vi "test_Open TCP connection using Initialize node.vi"(8 "error in (no error)":errorcluster, 11 "TestCase in":refnum<class "Ethernet Protocol Tests.lvclass">) -> (0 "error out":errorcluster, 3 "TestCase out":refnum<class "Ethernet Protocol Tests.lvclass">)   [LabVIEW 2019, in "Ethernet Protocol Tests.lvclass"]
uses:
  Ethernet Protocol Tests.lvclass
  TCP/TCP.lvclass
  TCP/TCP.lvclass/TCP.ctl
  Constants.vi
  <vilib>/addons/_JKI Toolkits/VI Tester/TestCase.llb/TestCase.lvclass
  C:/Program Files (x86)/National Instruments/LabVIEW 2019/vi.lib/addons/_JKI Toolkits/VI Tester/TestCase.llb/TestCase.lvclass
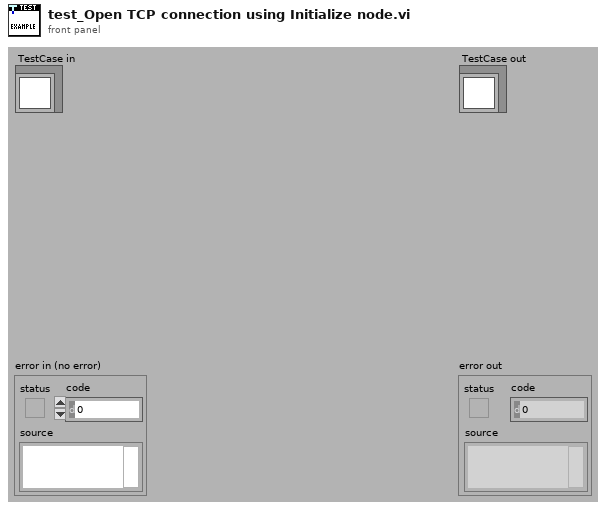
[diagram p1: front panel]
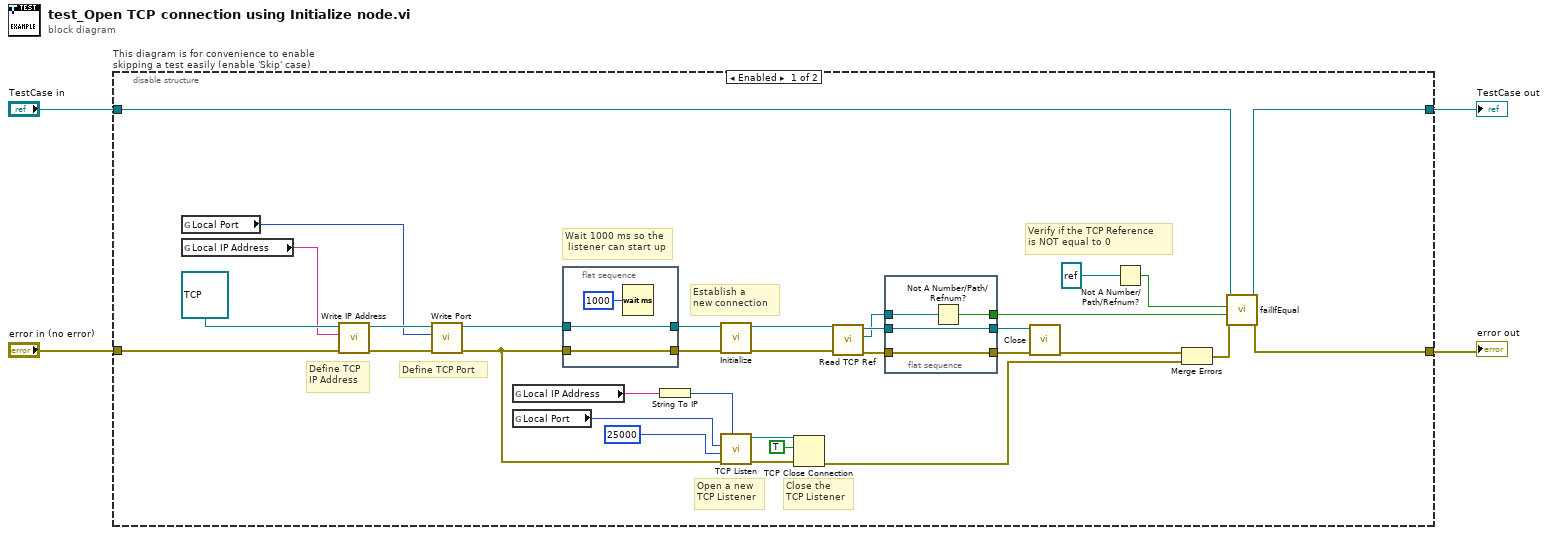
[diagram p0: block diagram]
diagram:
  n1 = disable-structure "This diagram is for convenience to enable skipping a test easily (enable 'Skip' case)" shown="Enabled" {
    disable-tunnel: "TestCase in" -> [w37 w48]
    disable-tunnel: [w25 w46] -> w1
    disable-tunnel: [w24 w47] -> w3
    disable-tunnel: "error in (no error)" -> [w33 w45]
    frame Enabled {
      # "Wait 1000 ms so the\n listener can start up"
      # "Verify if the TCP Reference \nis NOT equal to 0"
      # "Close the \nTCP Listener"
      # "Open a new \nTCP Listener"
      # "Establish a \nnew connection"
      # "Define TCP Port"
      # "Define TCP\nIP Address"
      n2 = global read "Constants.vi" "Local Port"() -> (w13:u16)
      n3 = global read "Constants.vi" "Local IP Address"() -> (w14:string)
      n4 = call "Write IP Address.vi"("error in (no error)"=w33, "IP Address"=w14, "Ethernet in"=refnum<class "TCP.lvclass"> refnum ("Protocols.lvlib:TCP.lvclass")) -> ("error out"=w35:errorcluster, "Ethernet out"=w36:refnum<class "TCP.lvclass">)  [unwired: 7 in]
      n5 = call "Write Port.vi"("error in (no error)"=w35, "Port"=w13, "Ethernet in"=w36) -> ("error out"=w17:errorcluster, "Ethernet out"=w16:refnum<class "TCP.lvclass">)  [unwired: 7 in]
      n6 = global read "Constants.vi" "Local IP Address"() -> (w12:string)
      n7 = global read "Constants.vi" "Local Port"() -> (w11:u16)
      n8 = flat-sequence {
        tunnel: w17 -> [w43]
        tunnel: [w43] -> w20
        tunnel: w16 -> [w42]
        tunnel: [w42] -> w18
        frame #0 {
          n9 = Wait (ms)(milliseconds to wait=u32 1000) -> ()  [unwired: 1 out]
        }
      }
      n10 = String To IP(1:w12) -> (0:w32:u32)
      n11 = call-dynamic "Initialize.vi"("error in (no error)"=w20, "Ethernet in"=w18) -> ("error out"=w19:errorcluster, "Ethernet out"=w15:refnum<class "TCP.lvclass">)  [unwired: 8 in]
      n12 = call <vilib>:"TCP Listen.vi"("net address"=w32, "error in (no error)"=w17, "timeout ms (wait forever: -1)"=25000, "port"=w11) -> ("error out"=w30:errorcluster, "connection ID"=w29:refnum<k5>)  [unwired: 3 in, 3 out]
      n13 = TCP Close Connection(connection ID=w29, abort (F)=TRUE, error in (no error)=w30) -> (error out=w27:errorcluster)  [unwired: 1 out]
      n14 = call "Read TCP Ref.vi"("error in (no error)"=w19, "Ethernet in"=w15) -> ("error out"=w10:errorcluster, "TCP Ref"=w5:refnum<k5>, "Ethernet out"=w8:refnum<class "TCP.lvclass">)  [unwired: 7 in]
      n15 = flat-sequence {
        tunnel: w10 -> [w41]
        tunnel: [w41] -> w9
        tunnel: w8 -> [w40]
        tunnel: [w40] -> w7
        tunnel: [w39] -> w6
        tunnel: w5 -> [w38]
        frame #0 {
          n16 = Not A Number/Path/Refnum?(number/path/refnum=w38) -> (NaN/Path/Refnum?=w39:bool)
        }
      }
      n17 = call-dynamic "Close.vi"("error in (no error)"=w9, "Ethernet in"=w7) -> ("error out"=w21:errorcluster)  [unwired: 8 in, 1 out]
      n18 = Not A Number/Path/Refnum?(number/path/refnum=refnum<k5> refnum ("TCP Ref")) -> (NaN/Path/Refnum?=w22:bool)
      n19 = Merge Errors(w21, w27) -> (w26:errorcluster)
      n20 = call-dynamic "failIfEqual.vi"("error in (no error)"=w26, "y"=w6, "x"=w22, "TestCase in"=w37) -> ("error out"=w24:errorcluster, "TestCase out"=w25:refnum<class "Ethernet Protocol Tests.lvclass">)  [unwired: 6 in]
    }
    frame Disabled {
      # "skip test result while test is under development"
      n21 = call <vilib>:"skip.vi"("error in (no error)"=w45, "TestCase in"=w48) -> ("error out"=w47:errorcluster, "TestCase out"=w46:refnum<class "Ethernet Protocol Tests.lvclass">)  [unwired: 8 in]
    }
  }
  "error out" <- w3
  "TestCase out" <- w1
